vi "Test Write Taus.vi"() -> ()   [LabVIEW 2012]
uses:
  Reusable/File IO/File Utilities.lvlib
panel:
  in  "Boolean":bool
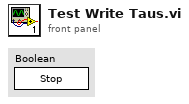
[diagram p1: front panel]
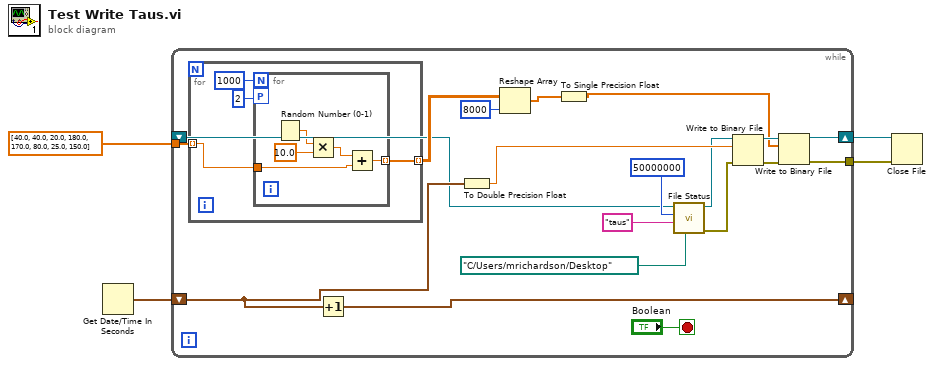
[diagram p0: block diagram]
diagram:
  n1 = Get Date/Time In Seconds() -> (seconds since 1Jan1904=w4:timestamp)
  n2 = while {
    shift-right: [w13] -> _
    shift-left: w4 -> [w12]
    tunnel: sgl[] [40.0, 40.0, 20.0, 180.0, 170.0, 80.0, 25.0, 150.0] -> [w14]
    tunnel: [w6] -> w1
    shift-right: [w7] -> w2
    shift-left: _ -> [w5]
    stop <- "Boolean" stop-if-true
    n3 = for {
      tunnel: w14 -> [w25] mode=indexing
      tunnel: [w24] -> w11 mode=indexing
      n4 = for {
        N: 1000 -> [_]
        workers-P: 2 -> [_]
        tunnel: w25 -> [w29]
        tunnel: [w28] -> w24 mode=indexing
        n5 = Random Number (0-1)() -> (number: 0 to 1=w32:dbl)
        n6 = Multiply(x=w32, y=10.0) -> (x*y=w30:dbl)
        n7 = Add(x=w30, y=w29) -> (x+y=w28:dbl)
      }
    }
    n8 = Increment(x=w12) -> (x+1=w13:timestamp)
    n9 = To Double Precision Float(number=w12) -> (double precision float=w23:dbl)
    n10 = Reshape Array(w11, 8000 ("dimension size")) -> (w9:dbl[])
    n11 = To Single Precision Float(number=w9) -> (single precision float=w8:sgl[])
    n12 = call "File Status.vi"("Data Path"=path "C:/Users/mrichardson/Desktop" ("file path (use dialog)"), "prefix"="taus", "fSize"=i64 50000000, "fileRefIn"=w5) -> ("error out"=w16:errorcluster, "fileRefOut"=w17:refnum<file>)  [unwired: 6 in]
    n13 = Write to Binary File(file (use dialog)=w17, data=w23, error in=w16) -> (refnum out=w21:refnum<file>, error out=w22:errorcluster)  [unwired: 3 in, 1 out]
    n14 = Write to Binary File(file (use dialog)=w21, data=w8, error in=w22) -> (refnum out=w7:refnum<file>, error out=w6:errorcluster)  [unwired: 3 in, 1 out]
  }
  n15 = Close File(refnum=w2, error in=w1) -> ()  [unwired: 2 out]
